vi "DrawRings.vi"(0 "Ring Array":cluster{"Radius":dbl, "a":dbl}[][](array[cluster]) {"a" format="%.2f"; "Radius" format="%.2f"}, 3 "a":dbl format="%.2f") -> (5 "ring locations (a)":string, 7 "flattened locations":string, 8 "Ring Pict":picture, 9 "rings (m)":dbl[](array[numeric]))   [LabVIEW 2022 SP3]
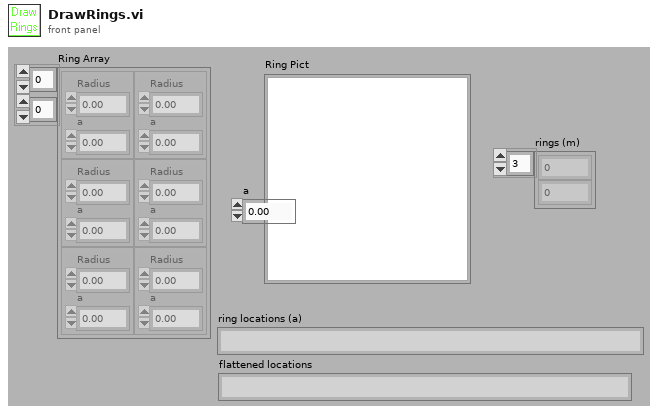
[diagram p1: front panel]
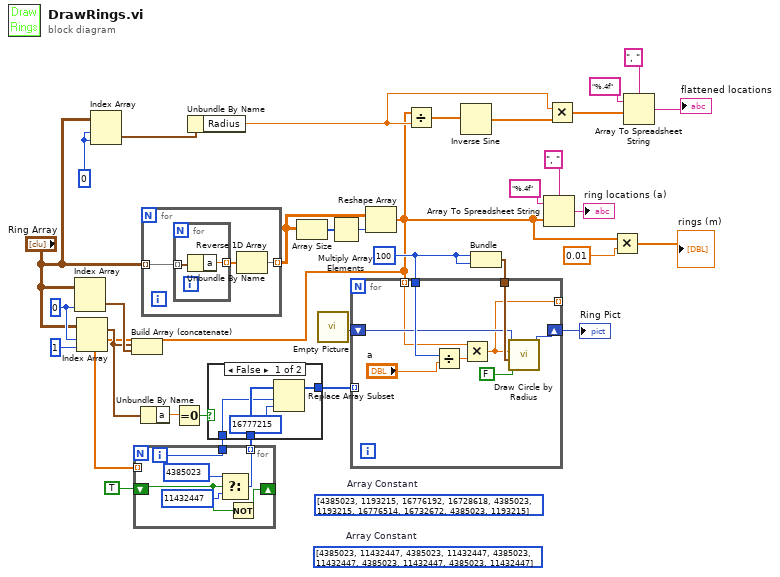
[diagram p0: block diagram]
diagram:
  w5 = 0
  (unwired) u32[] [4385023, 11432447, 4385023, 11432447, 4385023, 11432447, 4385023, 11432447, 4385023, 11432447]  # Array Constant
  (unwired) u32[] [4385023, 1193215, 16776192, 16728618, 4385023, 1193215, 16776514, 16732672, 4385023, 1193215]  # Array Constant
  w32 = 0
  w30 = 100
  n1 = Index Array(array="Ring Array", index (col)=w32) -> (element=w19:cluster{"Radius":dbl, "a":dbl}[])  [unwired: 1 in]
  n2 = Index Array(array="Ring Array", index (row)=w32, index (col)=1) -> (element=w7:cluster{"Radius":dbl, "a":dbl})
  n3 = Index Array(array="Ring Array", index (row)=w5, index (col)=w5) -> (element=w4:cluster{"Radius":dbl, "a":dbl})
  n4 = Build Array (concatenate)(w7, w19) -> ()  [unwired: 1 out]
  n5 = Unbundle By Name(w7) -> ("a"=w27:dbl)
  n6 = for {
    tunnel: "Ring Array" -> [w36] mode=indexing
    tunnel: [w34] -> w16 mode=indexing
    n7 = for {
      tunnel: w36 -> [w38] mode=indexing
      tunnel: [w37] -> w35 mode=indexing
      n8 = Unbundle By Name(w38) -> ("a"=w37:dbl)
    }
    n9 = Reverse 1D Array(array=w35) -> (reversed array=w34:dbl[])
  }
  n10 = Equal To 0?(x=w27) -> (x = 0?=w23:bool)
  n11 = Unbundle By Name(w4) -> ("Radius"=w12:dbl)
  n12 = Array Size(array=w16) -> (size(s)=w18:i32[])
  n13 = call "Empty Picture"() -> ("empty picture"=w31:picture)
  n14 = Multiply Array Elements(1:w18) -> (0:w17:i32)
  n15 = Reshape Array(w16, w17) -> (w3:dbl[])
  n16 = for {
    shift-right: [w41] -> _
    shift-left: TRUE -> [w42]
    tunnel: [w40] -> w25 mode=indexing
    tunnel: [w39] -> w24
    tunnel: w3 -> [_] mode=indexing
    i -> [w39]
    n17 = Select(t=u32 4385023, s=w42, f=u32 11432447) -> (s? t:f=w40:u32)
    n18 = Not(x=w42) -> (.not. x?=w41:bool)
  }
  n19 = case shown="False" w23 {
    tunnel: w25 -> [w48 w49]
    tunnel: [w47 w49] -> w15
    tunnel: w24 -> [w45 _]
    frame False {
      n20 = Replace Array Subset(array=w48, new element=u32 16777215, index=w45) -> (w47:u32[])
    }
    frame True {
    }
  }
  n21 = Divide(x=w3, y=w12) -> (x/y=w14:dbl[])
  n22 = Inverse Sine(1:w14) -> (0:w13:dbl[])
  n23 = Bundle(w30, w30) -> (w29:cluster{i32, i32})  [unwired: 1 out]
  n24 = for {
    tunnel: w29 -> [w57]
    shift-right: [w56] -> w28
    shift-left: w31 -> [w54]
    tunnel: w30 -> [w55]
    tunnel: [w53] -> _ mode=indexing
    tunnel: w3 -> [w50] mode=indexing
    tunnel: w15 -> [_] mode=indexing
    n25 = Divide(x=w55, y="a") -> (x/y=w58:dbl)
    n26 = Multiply(x=w50, y=w58) -> (x*y=w53:dbl)
    n27 = call <vilib>:"Draw Circle by Radius.vi"("fill?(F)"=FALSE, "pixel center"=w57, "radius"=w53, "picture"=w54) -> ("new picture"=w56:picture)  [unwired: 4 in, 3 out]
  }
  "Ring Pict" <- w28
  n28 = Array To Spreadsheet String(delimiter (Tab)=", ", array=w3, 3:"%.4f" ("format string")) -> (spreadsheet string=→"ring locations (a)":string)
  n29 = Multiply(x=w12, y=w13) -> (x*y=w9:dbl[])
  n30 = Multiply(x=w3, y=0.01) -> (x*y=→"rings (m)":dbl[])
  n31 = Array To Spreadsheet String(delimiter (Tab)=", ", array=w9, 3:"%.4f" ("format string")) -> (spreadsheet string=→"flattened locations":string)
